vi "Test Case Result Execution Time.vi"(8 "error in (no error)":errorcluster, 11 "Test Test Case Result In":refnum<class "Test Case Result Test.lvclass">) -> (0 "error out":errorcluster, 3 "Test Test Case Result Out":refnum<class "Test Case Result Test.lvclass">)   [LabVIEW 2020, in "LUnit Tests.lvlib" / "Test Case Result Test.lvclass"]
uses:
  Test Case Result Test.lvclass
  Test Dummys/Test Test Case/Test Test Case.lvclass
  source/Framework/Result Types/Case Result/Test Case Result.lvlib
  <vilib>/Astemes/LUnit/Test Case.lvclass
  C:/Git/astemes-lunit/source/Framework/Test Case/LUnit Test Case.lvclass
  C:/Program Files (x86)/National Instruments/LabVIEW 2020/vi.lib/Astemes/LUnit/Test Case.lvclass
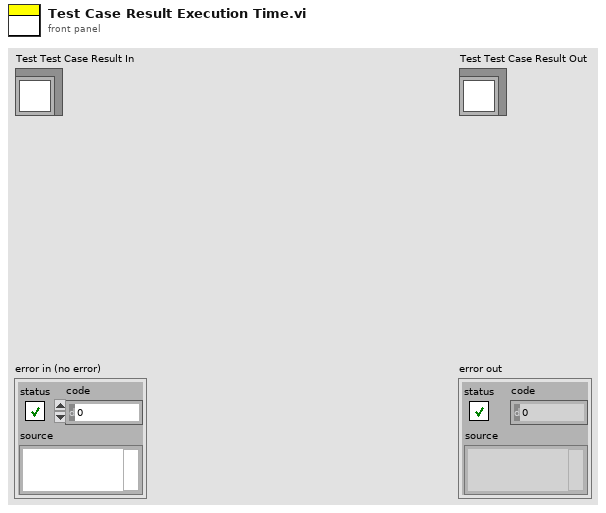
[diagram p1: front panel]
types:
  T1 = typedef "Test Case Result.lvlib/Test Case Result.ctl" = map{string, T2}
  T2 = typedef "Method Result.lvlib/Method Result.ctl" = cluster{"Test Case":string, "Test Method Name":string, "Status":T3, "Assertion Results":T4[], "Execution time":dbl, "Result String":string}
  T3 = typedef "Assertion Result.lvlib/Status.ctl" = enum16{"Pass", "Fail", "Error", "Skipped", "Setup Error", "Broken", "Teardown Error"}
  T4 = typedef "Assertion Result.lvlib/Assertion Result.ctl" = cluster{"Status":T3, "Message":string, "Description":string, "Assertion Type":T5}
  T5 = typedef "Assertion Result.lvlib/Assertion Type.ctl" = enum16{"None", "Pass", "Fail", "Skip", "Pass if Equal", "Fail if Equal", "Pass if Error", "Fail if Error", "Pass if", "Fail if"}
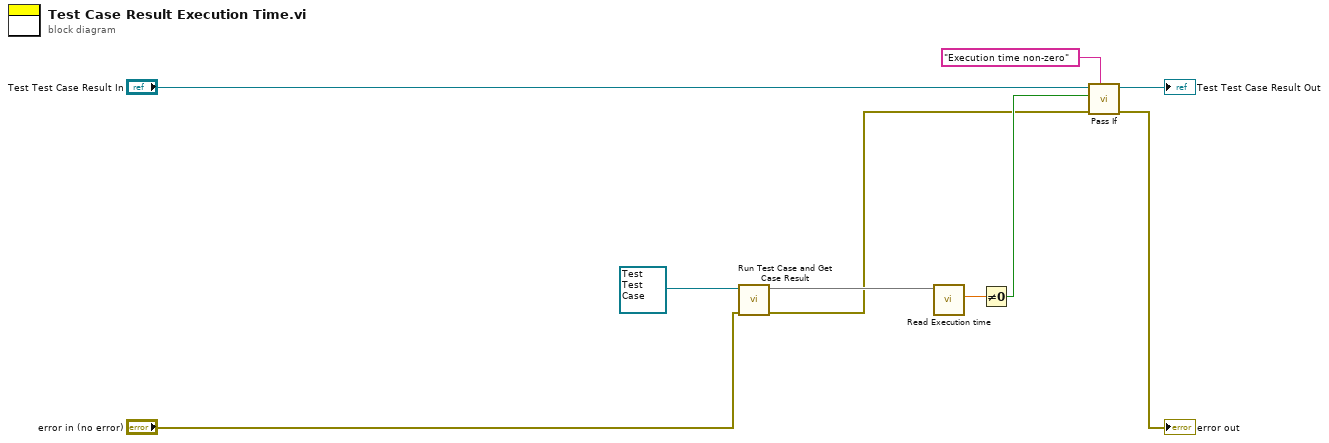
[diagram p0: block diagram]
diagram:
  n1 = call "Run Test Case and Get Case Result.vi"("error in (no error)"="error in (no error)", "Error First Test Case in"=refnum<class "Test Test Case.lvclass"> refnum ("Test Test Case.lvclass")) -> ("error out"=w1:errorcluster, "Test Case Result out"=w4:T1)  [unwired: 8 in]
  n2 = call "Read Execution time.vi"("Test Case Result In"=w4) -> ("Execution time"=w6:dbl)  [unwired: 9 in, 1 out]
  n3 = Not Equal To 0?(x=w6) -> (x != 0?=w5:bool)
  n4 = call <vilib>:"Pass If.vi"("Description"="Execution time non-zero", "error in (no error)"=w1, "Pass?"=w5, "LUnit Test Case In"="Test Test Case Result In") -> ("error out"=→"error out":errorcluster, "LUnit Test Case Out"=→"Test Test Case Result Out":refnum<class "Test Case Result Test.lvclass">)  [unwired: 6 in]
